vi "Add Sequence.vi"(8 "error in (no error)":errorcluster, 10 "Sequence In":refnum<class "Sequence.lvclass">, 11 "Mediator in":refnum<class "Mediator.lvclass">) -> (0 "error out":errorcluster, 3 "Mediator out":refnum<class "Mediator.lvclass">)   [LabVIEW 2015, in "Mediator.lvlib" / "Mediator.lvclass"]
doc: "Adds a Sequence to the Mediator. If the Mediator is idle the sequence will execute immediately. If the Mediator is currently processing another sequence this will add it to the queue to be run."
uses:
  Mediator.lvclass
  Sequence/Sequence.lvclass
  Mediator.lvclass/Mediator.ctl
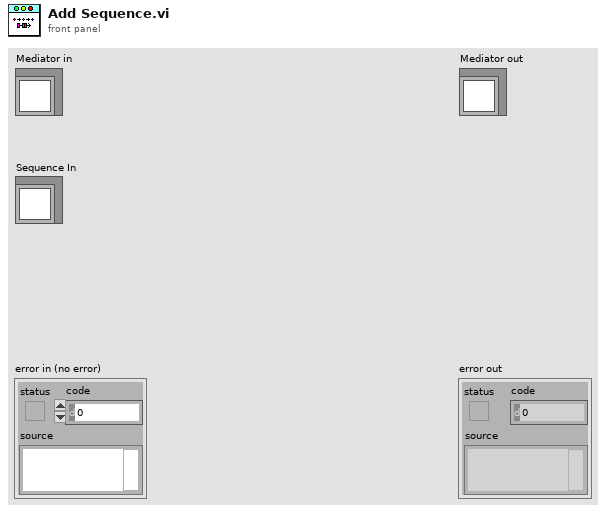
[diagram p1: front panel]
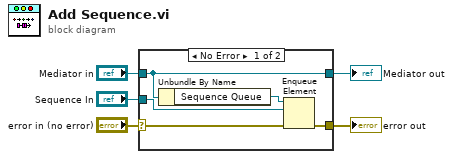
[diagram p0: block diagram]
diagram:
  n1 = case shown="No Error" "error in (no error)" {
    selector: "error in (no error)" -> [w7 w12]
    tunnel: [w6 w12] -> w4
    tunnel: [w10 w11] -> w2
    tunnel: "Mediator in" -> [w10 w11]
    tunnel: "Sequence In" -> [w8 _]
    frame No Error {
      n2 = Unbundle By Name(w10) -> ("Sequence Queue"=w9:refnum<queue>)
      n3 = Enqueue Element(queue=w9, element=w8, error in (no error)=w7) -> (error out=w6:errorcluster)  [unwired: 1 in, 2 out]
    }
    frame Error {
    }
  }
  "error out" <- w4
  "Mediator out" <- w2
